vi "Measurement Logic.vi"() -> ()   [LabVIEW 2022 SP3, in "Acoustic Calibration.lvlib"]
uses:
  Acoustic Calibration.lvlib
  <vilib>/Plug-In SDKs/Measurements/Measure Call Context/Measure Call Context.lvclass
  Measurement Configuration.ctl
  Measurement Results.ctl
  <vilib>/gRPC/Generated APIs/ni/protobuf/types/RPC Messages/ni_protobuf_types_DoubleXYData.ctl
  <vilib>/gRPC/Generated APIs/ni/protobuf/types/ni.protobuf.types.lvlib
panel:
  out "measurement results":T1={"xy data out"={"x_data"=[], "y_data"=[]}, "double array out"=[0.0], "double out"=0.0, "U32 array out"=[0], "U32 out"=0, "U64 array out"=[0], "U64 out"=0, "I32 array out"=[0], "I32 out"=0, "I64 array out"=[0], "I64 out"=0, "bool out"=FALSE, "string out"="Empty", "u32 color ring out"=0, "u32 animal enum out"=enum."Rabbit"} {"u32 color ring out" items=["Red", "Green", "Blue"]}
  in  "measurement configuration":T3={"double array in"=[3.4, 5.6], "double in"=1.2, "U32 array in"=[32, 33], "U32 in"=32, "U64 array in"=[64, 65], "U64 in"=64, "I32 array in"=[-32, -33], "I32 in"=-32, "I64 array in"=[-64, -65], "I64 in"=-64, "bool in"=TRUE, "string in"="Lorem ipsum dolor sit", "u32 color ring in"=1, "u32 animal enum in"=enum."Gopher"} {"u32 color ring in" items=["Red", "Green", "Blue"]}
  out "measure call context out":refnum<class "Measure Call Context.lvclass">
  in  "measure call context in":refnum<class "Measure Call Context.lvclass">
  out "error out":errorcluster
  in  "error in":errorcluster
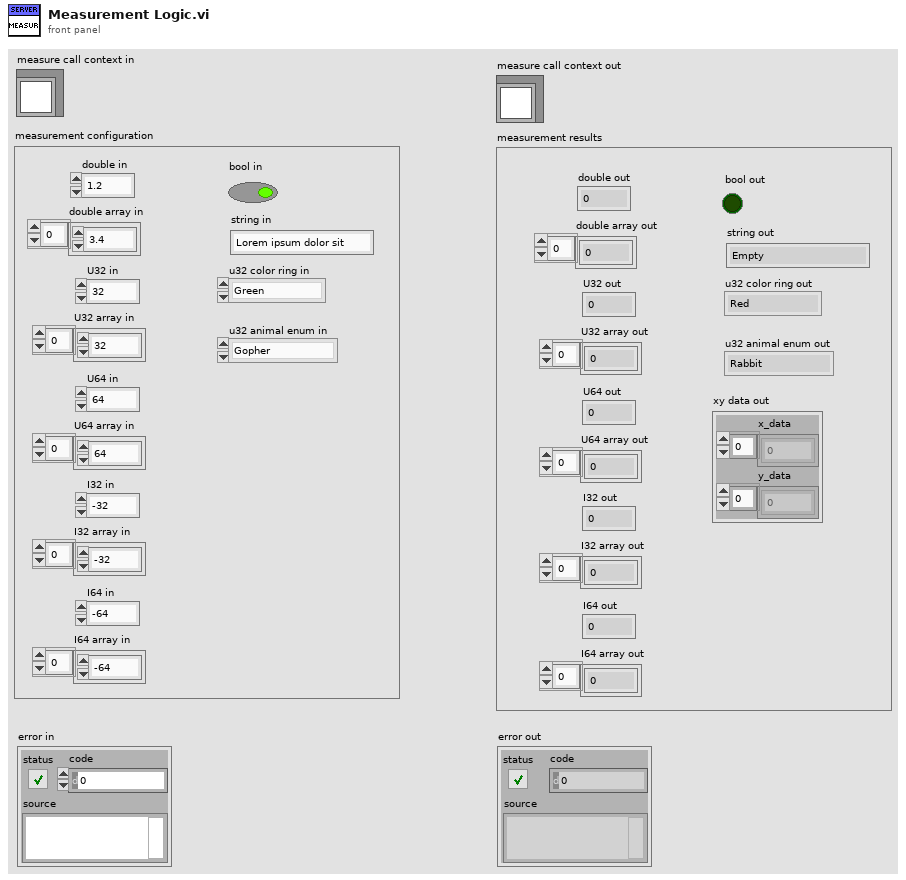
[diagram p1: front panel]
types:
  T1 = typedef "Acoustic Calibration.lvlib/Measurement Results.ctl" = cluster{"xy data out":T2, "double array out":dbl[], "double out":dbl, "U32 array out":u32[], "U32 out":u32, "U64 array out":u64[], "U64 out":u64, "I32 array out":i32[], "I32 out":i32, "I64 array out":i64[], "I64 out":i64, "bool out":bool, "string out":string, "u32 color ring out":u32, "u32 animal enum out":enum32{"Rabbit", "Gopher", "Badger"}}
  T2 = typedef "ni.protobuf.types.lvlib/ni_protobuf_types_DoubleXYData.ctl" = cluster{"x_data":dbl[], "y_data":dbl[]}
  T3 = typedef "Acoustic Calibration.lvlib/Measurement Configuration.ctl" = cluster{"double array in":dbl[], "double in":dbl, "U32 array in":u32[], "U32 in":u32, "U64 array in":u64[], "U64 in":u64, "I32 array in":i32[], "I32 in":i32, "I64 array in":i64[], "I64 in":i64, "bool in":bool, "string in":string, "u32 color ring in":u32, "u32 animal enum in":enum32{"Rabbit", "Gopher", "Badger"}}
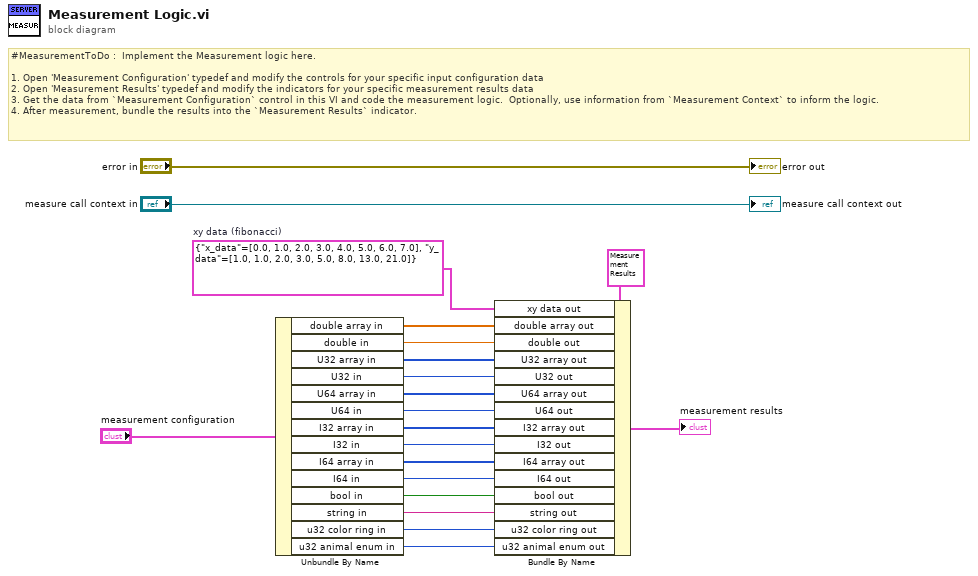
[diagram p0: block diagram]
diagram:
  w3 = T2 {"x_data"=[0.0, 1.0, 2.0, 3.0, 4.0, 5.0, 6.0, 7.0], "y_data"=[1.0, 1.0, 2.0, 3.0, 5.0, 8.0, 13.0, 21.0]}  # xy data (fibonacci)
  # "#MeasurementToDo :  Implement the Measurement logic here.\n\n1. Open 'Measurement Configuration' typedef and modify the controls for your specific input configuration data\n2. Open 'Measurement Results' typedef and modify the indicators for your specific measurement results data\n3. Get the data from `Measurement Configuration` control in this VI and code the measurement logic.  Optionally, use information from `Measurement Context` to inform the logic.\n4. After measurement, bundle the results into the `Measurement Results` indicator."
  n1 = Unbundle By Name("measurement configuration") -> ("double array in"=w17:dbl[], "double in"=w16:dbl, "U32 array in"=w15:u32[], "U32 in"=w14:u32, "U64 array in"=w13:u64[], "U64 in"=w12:u64, "I32 array in"=w11:i32[], "I32 in"=w10:i32, "I64 array in"=w9:i64[], "I64 in"=w8:i64, "bool in"=w7:bool, "string in"=w6:string, "u32 color ring in"=w5:u32, "u32 animal enum in"=w4:enum32{"Rabbit", "Gopher", "Badger"})
  n2 = Bundle By Name(cluster=T1 {"xy data out"={"x_data"=[], "y_data"=[]}, "double array out"=[], "double out"=0.0, "U32 array out"=[0], "U32 out"=0, "U64 array out"=[0], "U64 out"=0, "I32 array out"=[0], "I32 out"=0, "I64 array out"=[0], "I64 out"=0, "bool out"=FALSE, "string out"="Empty", "u32 color ring out"=0, "u32 animal enum out"=enum."Rabbit"} ("Measurement Results"), "xy data out"=w3, "double array out"=w17, "double out"=w16, "U32 array out"=w15, "U32 out"=w14, "U64 array out"=w13, "U64 out"=w12, "I32 array out"=w11, "I32 out"=w10, "I64 array out"=w9, "I64 out"=w8, "bool out"=w7, "string out"=w6, "u32 color ring out"=w5, "u32 animal enum out"=w4) -> (→"measurement results":T1)
  "error out" <- "error in"
  "measure call context out" <- "measure call context in"
